vi "Adv_GetXMLFromSPE.vi"(8 "error in (no error)":errorcluster, 11 "Path In":path) -> (0 "error out":errorcluster, 2 "XML":string, 3 "SPE Refnum":refnum<file>)   [LabVIEW 2018, in "LightField Automation.lvclass"]
uses:
  LightField Automation.lvclass
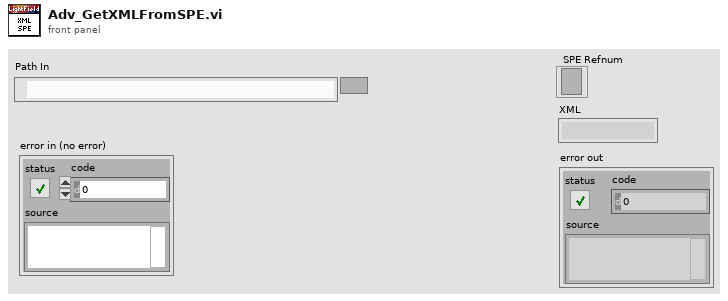
[diagram p1: front panel]
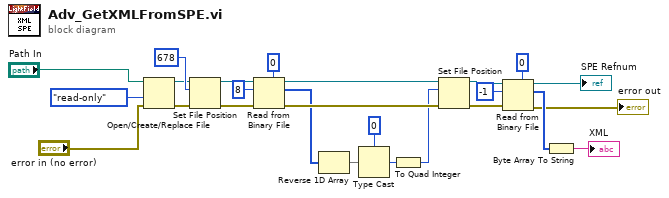
[diagram p0: block diagram]
diagram:
  n1 = Open/Create/Replace File(file path (use dialog)="Path In", error in="error in (no error)", access (0:read/write)=enum16{"read/write", "read-only", "write-only"}."read-only") -> (refnum out=w20:refnum<file>, error out=w21:errorcluster)  [unwired: 3 in, 1 out]
  n2 = Set File Position(offset (in bytes) (0)=i64 678, refnum=w20, error in=w21) -> (refnum out=w16:refnum<file>, error out=w17:errorcluster)  [unwired: 1 in]
  n3 = Read from Binary File(5:u8 0, 8:w17, 10:8 ("count (1)"), 11:w16) -> (0:w25:errorcluster, 2:w23:u8[], 3:w24:refnum<file>)  [unwired: 2 in, 1 out]
  n4 = Reverse 1D Array(array=w23) -> (reversed array=w8:u8[])
  n5 = Type Cast(type=u64 0, x=w8) -> (*(type *) &x=w13:u64)
  n6 = To Quad Integer(1:w13) -> (0:w14:i64)
  n7 = Set File Position(offset (in bytes) (0)=w14, refnum=w24, error in=w25) -> (refnum out=w12:refnum<file>, error out=w11:errorcluster)  [unwired: 1 in]
  n8 = Read from Binary File(5:u8 0, 8:w11, 10:-1 ("count (1)"), 11:w12) -> (0:→"error out":errorcluster, 2:w15:u8[], 3:→"SPE Refnum":refnum<file>)  [unwired: 2 in, 1 out]
  n9 = Byte Array To String(unsigned byte array=w15) -> (string=→"XML":string)
